vi "solar_write ThisHS.vi"(8 "error in (no error)":errorcluster, 10 "CMD_DATA":variant, 11 "solar in":refnum<class "solar.lvclass">) -> (0 "error out":errorcluster, 3 "solar out":refnum<class "solar.lvclass">)   [LabVIEW 2018, in "solar.lvclass"]
doc: "This sets the command data variant that contains the Handshake variant attribute to respond to the calling target."
uses:
  solar.lvclass
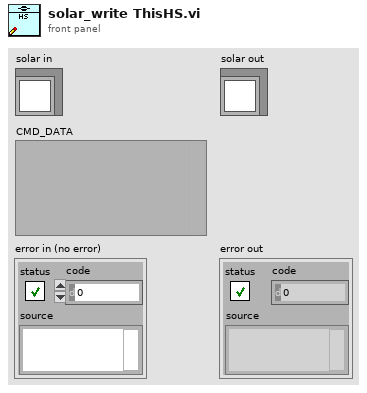
[diagram p1: front panel]
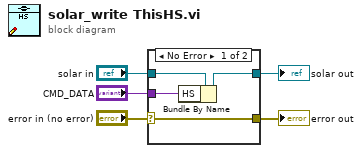
[diagram p0: block diagram]
diagram:
  n1 = case shown="No Error" "error in (no error)" {
    selector: "error in (no error)" -> [w6 w11]
    tunnel: "solar in" -> [w9 w10]
    tunnel: [w8 w10] -> w4
    tunnel: "CMD_DATA" -> [w7 _]
    tunnel: [w6 w11] -> w2
    frame No Error {
      n2 = Bundle By Name(cluster=w9, "HS"=w7) -> (w8:refnum<class "solar.lvclass">)
    }
    frame Error {
    }
  }
  "error out" <- w2
  "solar out" <- w4
